vi "Flatten Value.vi"(8 "Error In":errorcluster, 11 "Bool Array In":refnum<class "1D Bool.lvclass">) -> (0 "Error Out":errorcluster, 1 "Value":string, 3 "Bool Array Out":refnum<class "1D Bool.lvclass">)   [LabVIEW 2020, in "NI_VIAnCFGDataStructure.lvlib" / "1D Bool.lvclass"]
uses:
  <vilib>/addons/analyzer/VIAnCFGDataStructure/Data Types/Bool Array/1D Bool.lvclass
  <vilib>/addons/analyzer/VIAnCFGDataStructure/Data Types/Bool Array/1D Bool.lvclass/1D Bool.ctl
  <vilib>/addons/analyzer/VIAnCFGDataStructure/Tree Manager/Tree.lvclass
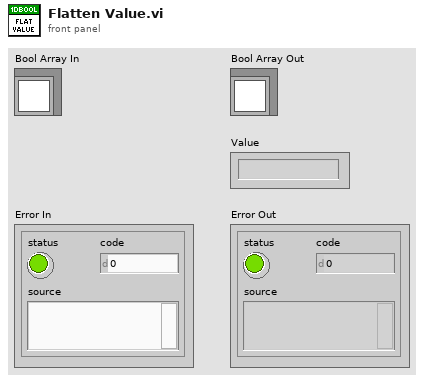
[diagram p1: front panel]
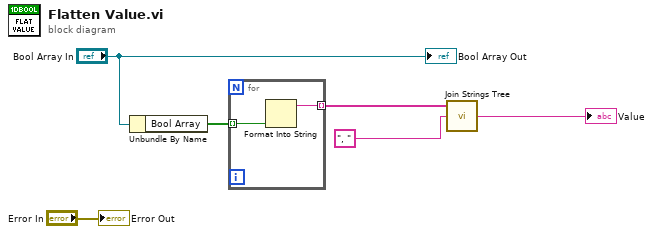
[diagram p0: block diagram]
diagram:
  n1 = Unbundle By Name("Bool Array In") -> ("Bool Array"=w5:bool[])
  n2 = for {
    tunnel: w5 -> [w8] mode=indexing
    tunnel: [w7] -> w3 mode=indexing
    n3 = Format Into String(w8) -> (resulting string=w7:string)  [unwired: 3 in, 1 out]
  }
  n4 = call <vilib>:"Join Strings Tree.vi"("Separator (,)"=", ", "Strings In"=w3) -> ("String"=→"Value":string)  [unwired: 1 in]
  "Bool Array Out" <- "Bool Array In"
  "Error Out" <- "Error In"
